vi "Open and Run VI (using Static Ref).vi"(6 "State (Hidden)":T1(ring)=enum."Hidden", 8 "error in (no error)":errorcluster, 10 "Run? (T)":bool=TRUE, 11 "Static VI reference":refnum<vi>) -> (0 "error out":errorcluster, 2 "Front Panel Window Was Open?":bool, 3 "VI":refnum<vi>)   [LabVIEW 2015, in "Utility.lvlib"]
doc: "This VI is used to dynamically open and run (if desired) another VI.\n\nThe initial state of the window can be specified (defaults to hidden).\n\nNote: this VI should normally be used in conjunction with a static VI reference passed in from the parent VI. This method causes the target VI to automatically be included in the build, and also seems to offer better performace starting the VI. Another benefit is that a hard-coded path does not need to be used."
uses:
  Utility.lvlib
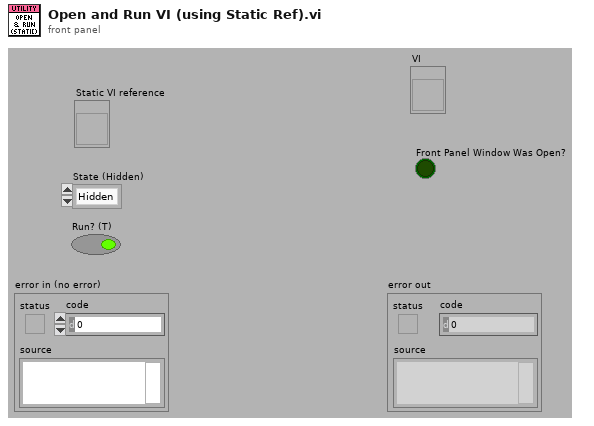
[diagram p1: front panel]
types:
  T1 = enum32{"Invalid", "Standard", "Closed", "Hidden", "Minimized", "Maximized"}
  T2 = enum32{"Bad", "Idle", "Run top level", "Running"}
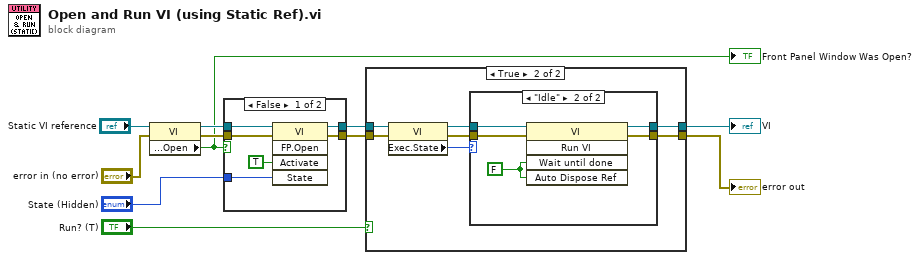
[diagram p0: block diagram]
diagram:
  n1 = property class="VI"(reference="Static VI reference", error in="error in (no error)") -> (reference out=w5:refnum<vi>, error out=w4:errorcluster, "Front Panel.Open"=w3:bool)
  "Front Panel Window Was Open?" <- w3
  n2 = case shown="False" w3 {
    tunnel: "State (Hidden)" -> [w16 _]
    tunnel: [w15 w19] -> w10
    tunnel: [w14 w18] -> w9
    tunnel: w5 -> [w13 w19]
    tunnel: w4 -> [w12 w18]
    frame False {
      n3 = invoke class="VI" method="FP.Open"(reference=w13, error in=w12, "Activate"=TRUE ("Activate?"), "State"=w16) -> (reference out=w15:refnum<vi>, error out=w14:errorcluster)  [unwired: 1 in, 3 out]
    }
    frame True {
    }
  }
  n4 = case shown="True" "Run? (T)" {
    tunnel: w10 -> [w21 w26]
    tunnel: w9 -> [w20 w24]
    tunnel: [w20 w28] -> w8
    tunnel: [w21 w27] -> w7
    frame False {
    }
    frame True {
      n5 = property class="VI"(reference=w26, error in=w24) -> (reference out=w25:refnum<vi>, error out=w23:errorcluster, "Exec.State"=w22:T2)
      n6 = case shown="\"Idle\"" w22 {
        tunnel: [w29 w35] -> w28
        tunnel: [w30 w33] -> w27
        tunnel: w25 -> [w30 w32]
        tunnel: w23 -> [w29 w31]
        frame Default {
          # "Cannot run VI\n(perhaps it is already running)"
        }
        frame "Idle" {
          w34 = FALSE ("Wait Until Done")
          n7 = invoke class="VI" method="Run VI"(reference=w32, error in=w31, "Wait until done"=w34, "Auto Dispose Ref"=w34) -> (reference out=w33:refnum<vi>, error out=w35:errorcluster)  [unwired: 1 in, 3 out]
        }
      }
    }
  }
  "VI" <- w7
  "error out" <- w8
